vi "gmmregTransform.vi"(0 "param0":dbl[](array[numeric]), 2 "ctrlPts":dbl[][](array[numeric]), 3 "pts":dbl[][](array[numeric]), 4 "normParams":dbl[](array[numeric]), 8 "denormParams":dbl[](array[numeric])) -> (7 "out":dbl[][](array[numeric]))   [LabVIEW 2017]
panel:
  out "denormParams out":dbl[](array[numeric])
  out "normParams out":dbl[](array[numeric])
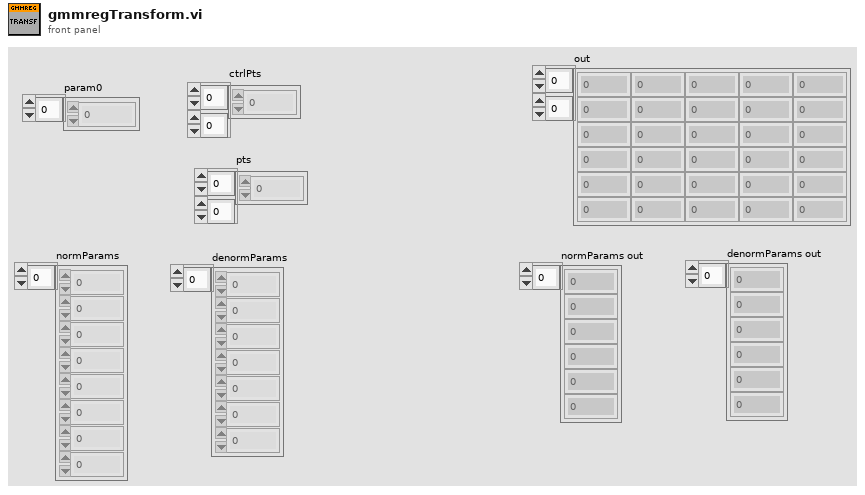
[diagram p1: front panel]
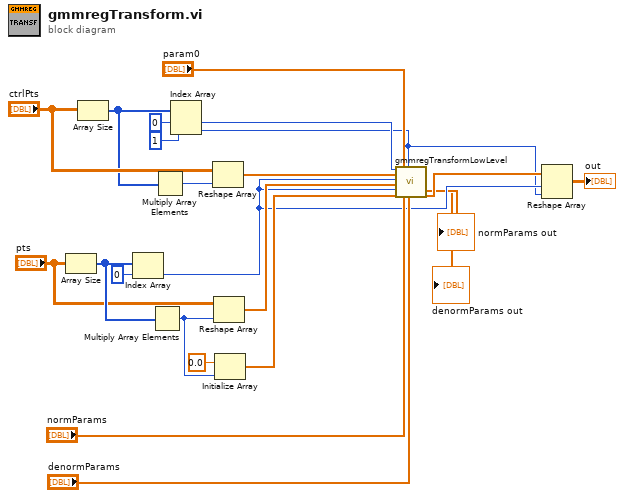
[diagram p0: block diagram]
diagram:
  n1 = Array Size(array="pts") -> (size(s)=w17:i32[])
  n2 = Array Size(array="ctrlPts") -> (size(s)=w20:i32[])
  n3 = Index Array(array=w17, index=0) -> (element=w5:i32)
  n4 = Multiply Array Elements(1:w17) -> (0:w15:i32)
  n5 = Multiply Array Elements(1:w20) -> (0:w19:i32)
  n6 = Index Array(array=w20, index #1=0 ("index"), index #2=1 ("index")) -> (element #1=w12:i32, element #2=w4:i32)
  n7 = Reshape Array("ctrlPts", w19) -> (w11:dbl[])
  n8 = Reshape Array("pts", w15) -> (w10:dbl[])
  n9 = Initialize Array(0.0 ("element"), w15) -> (w9:dbl[])
  n10 = call "gmmregTransformLowLevel.vi"("nctrlpts"=w12, "coordCtrlPts"=w11, "npts"=w5, "coord"=w10, "nout"=w5, "out"=w9, "param0"="param0", "normParams"="normParams", "dim"=w4, "denormParams"="denormParams") -> ("denormParams out"=→"denormParams out":dbl[], "normParams out"=→"normParams out":dbl[], "out out"=w6:dbl[])  [unwired: 4 in, 3 out]
  n11 = Reshape Array(w6, w5, w4) -> (→"out":dbl[][])
